vi "Open_File_from_Folder.vi"(0 "path name":string, 1 "prompt":string, 2 "pattern label":string, 3 "pattern (all files)":string, 4 "App Path":path) -> (5 "selected path":path, 6 "cancelled":bool)   [LabVIEW 2011]
doc: "This VI is an extension of a normal \"File Dialog\" box. It includes error checking for canceling the file selection process. It also forces the name and location of the start path. The start path is one level above the application path. If this path does not exist it will create it.\n\nThis VI is very convenient if you want to lock the name and location of paths for data files in your application. This removes a little flexibility from the user but greatly simplifies writing and debugging the application.\n\nPattern - Enter \"*.txt\" if you want to limit the pattern to text files. Use a semicolon to use multiple patterns. For example, enter \"*.csv;*.txt\" for text and csv files.\n\nPattern label - this will appear in the dialog box. So if the pattern is \"*.txt\" the pattern label should be \"Text Files\"\n\nPrompt - appears at top of dialog box. For example \"Open PGA309 Data File\"\n\nApp Path - connect to the \"current vi path\".\n\nPath name - name of the path you want to save or load from. For example \"\\PGA309_DATA\" would open this folder if it exists. If it does not exist, it will create it.\n\nSelected path - the path and file name of the file selected.\n\nCanceled - if the cancel button was pressed this is true."
panel:
  # "Input"
  # "Output"
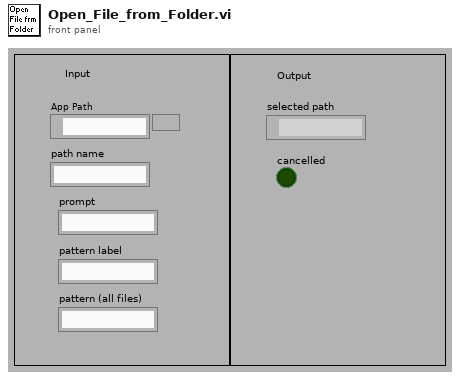
[diagram p1: front panel]
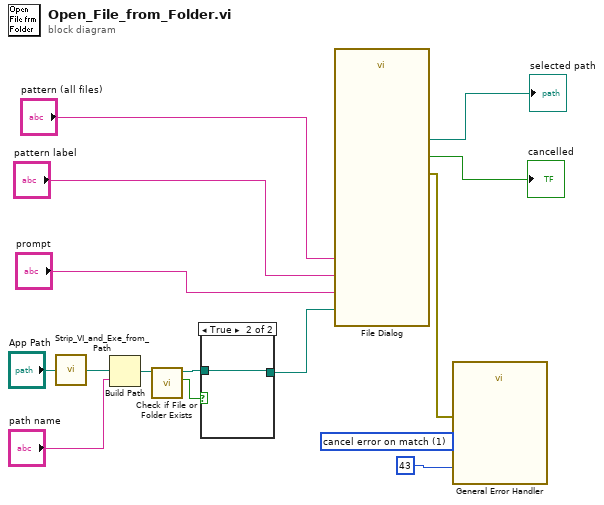
[diagram p0: block diagram]
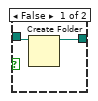
[diagram p2: hidden frame]
diagram:
  w8 = 1 items=["no exception", "cancel error on match", "set error on match"] ("[exception action] (none:0)")
  n1 = call "Strip_VI_and_Exe_from_Path.vi"("App Path"="App Path") -> ("App Path out"=w12:path)
  n2 = Build Path(base path=w12, name or relative path="path name") -> (appended path=w13:path)
  n3 = call <vilib>:"Check if File or Folder Exists.vi"("path"=w13) -> ("file or folder exists?"=w14:bool, "dup path"=w15:path)  [unwired: 8 in, 1 out]
  n4 = case shown="True" w14 {
    tunnel: w15 -> [w17 w18]
    tunnel: [w16 w18] -> w7
    frame False {
      n5 = Create Folder(path (use dialog)=w17) -> (created path=w16:path)  [unwired: 2 in, 2 out]
    }
    frame True {
    }
  }
  n6 = call "File Dialog"("start path"=w7, "prompt"="prompt", "pattern (all files)"="pattern (all files)", "pattern label"="pattern label") -> ("selected path"=→"selected path":path, "cancelled"=→"cancelled":bool, "error out"=w10:errorcluster)  [unwired: 8 in, 1 out]
  n7 = call <vilib>:"General Error Handler.vi"("error in (no error)"=w10, "[exception action] (none:0)"=w8, "[exception code]"=43) -> ()  [unwired: 8 in, 5 out]
